vi "Tetra_RxGain.vi"(0 "COMPORT":refnum<visa-resource-name>="COM4", 5 "error in (no error)":errorcluster, 6 "Open Ser(t)":bool, 7 "RXPORT(num)":i32=1 min=1 max=8 step=1, 8 "Close Ser(t)":bool, 9 "GAIN(code)":i32 min=0 max=7 step=1, 11 "REVC(T)":bool=TRUE, 13 "RO(t)":bool) -> (10 "vga(rxport)":string, 12 "gain code(value)":dbl, 14 "comport":refnum<visa-resource-name>="COM4", 16 "Readback (1-4)":i32[](array[numeric]), 19 "error out":errorcluster)   [LabVIEW 2018]
panel:
  out "revcVGA":i32
  out "cmd":string
  out "Success":bool
  out "concatenated string":string
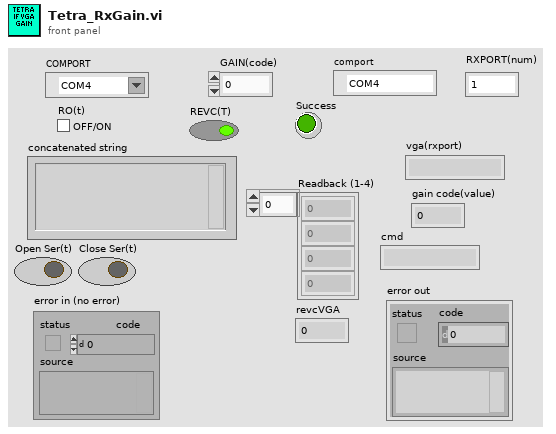
[diagram p1: front panel]
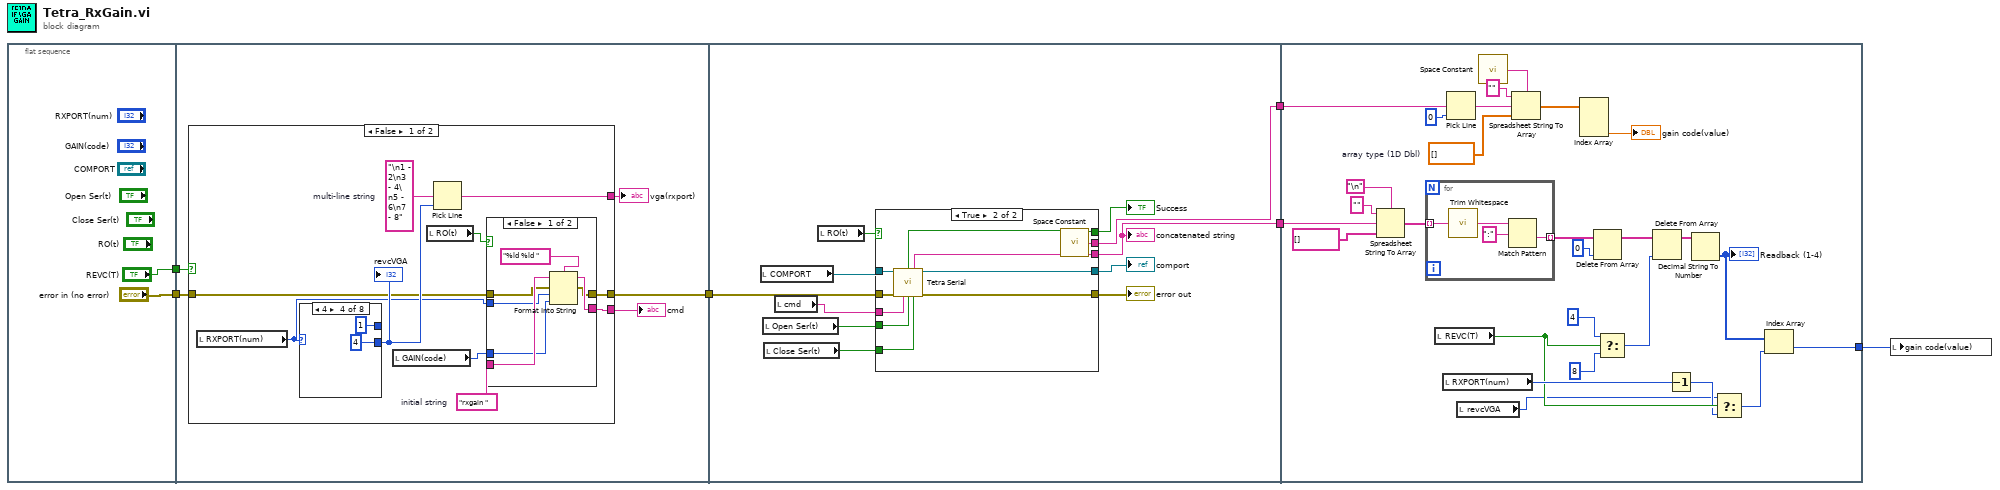
[diagram p0: block diagram]
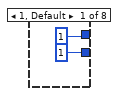
[diagram p3: hidden frame]
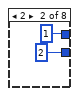
[diagram p4: hidden frame]
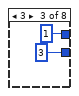
[diagram p5: hidden frame]
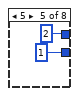
[diagram p6: hidden frame]
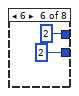
[diagram p7: hidden frame]
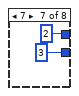
[diagram p8: hidden frame]
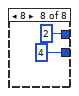
[diagram p9: hidden frame]
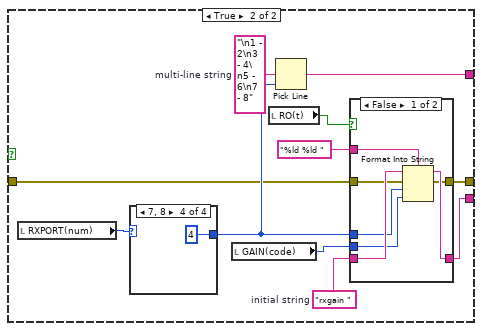
[diagram p10: hidden frame]
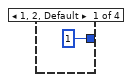
[diagram p12: hidden frame]
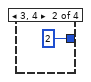
[diagram p13: hidden frame]
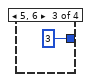
[diagram p14: hidden frame]
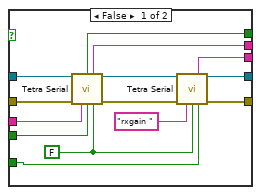
[diagram p15: hidden frame]
diagram:
  n1 = flat-sequence {
    tunnel: ["error in (no error)"] -> w3
    tunnel: ["REVC(T)"] -> w2
    tunnel: [w13] -> w6
    tunnel: w3 -> [w11]
    tunnel: w2 -> [w10]
    tunnel: w6 -> [w79]
    tunnel: [w80] -> w5
    tunnel: [w78] -> w4
    tunnel: w5 -> [w133]
    tunnel: w4 -> [w134]
    tunnel: [w112] -> w1
    frame #0 {
    }
    frame #1 {
      n2 = case shown="False" w10 {
        tunnel: [w23 w59] -> w9
        tunnel: [w22 w58] -> w13
        tunnel: [w19 w54] -> w12
        tunnel: w11 -> [w15 w49]
        frame False {
          w20 = "\n1 - 2\n3 - 4\n5 - 6\n7 - 8"  # multi-line string
          w21 = "rxgain "  # initial string
          n3 = local read "RXPORT(num)"() -> (w14:i32)
          n4 = case shown="4" w14 {
            tunnel: [1 ("RXPORT(num)") 2 ("RXPORT(num)") 3 ("RXPORT(num)") 4 ("RXPORT(num)") 1 ("RXPORT(num)") 2 ("RXPORT(num)") 3 ("RXPORT(num)") 4 ("RXPORT(num)")] -> w18
            tunnel: [1 ("RXPORT(num)") 1 ("RXPORT(num)") 1 ("RXPORT(num)") 1 ("RXPORT(num)") 2 ("RXPORT(num)") 2 ("RXPORT(num)") 2 ("RXPORT(num)") 2 ("RXPORT(num)")] -> _
            frame 1, Default {
            }
            frame 2 {
            }
            frame 3 {
            }
            frame 4 {
            }
            frame 5 {
            }
            frame 6 {
            }
            frame 7 {
            }
            frame 8 {
            }
          }
          "revcVGA" <- w18
          n5 = local read "GAIN(code)"() -> (w16:i32)
          n6 = local read "RO(t)"() -> (w17:bool)
          n7 = Pick Line(multi-line string=w20, line index=w18) -> (output string=w19:string)  [unwired: 1 in]
          n8 = case shown="False" w17 {
            tunnel: [w30 w32] -> w23
            tunnel: w21 -> [w29 w32]
            tunnel: w16 -> [w28 _]
            tunnel: w15 -> [w27 w31]
            tunnel: [w26 w31] -> w22
            tunnel: w14 -> [w24 _]
            frame False {
              n9 = Format Into String(format string="%ld %ld ", initial string=w29, error in=w27, w24, w28) -> (resulting string=w30:string, error out=w26:errorcluster)
            }
            frame True {
            }
          }
        }
        frame True {
          w55 = "\n1 - 2\n3 - 4\n5 - 6\n7 - 8"  # multi-line string
          w56 = "rxgain "  # initial string
          n10 = local read "RXPORT(num)"() -> (w51:i32)
          n11 = case shown="7, 8" w51 {
            tunnel: [1 ("RXPORT(num)") 2 ("RXPORT(num)") 3 ("RXPORT(num)") 4 ("RXPORT(num)")] -> w53
            frame 1, 2, Default {
            }
            frame 3, 4 {
            }
            frame 5, 6 {
            }
            frame 7, 8 {
            }
          }
          n12 = local read "GAIN(code)"() -> (w50:i32)
          n13 = local read "RO(t)"() -> (w52:bool)
          n14 = Pick Line(multi-line string=w55, line index=w53) -> (output string=w54:string)  [unwired: 1 in]
          n15 = case shown="False" w52 {
            tunnel: "%ld %ld " -> [w66 _]
            tunnel: [w65 w68] -> w59
            tunnel: w56 -> [w64 w68]
            tunnel: w50 -> [w63 _]
            tunnel: w53 -> [w62 _]
            tunnel: w49 -> [w61 w67]
            tunnel: [w60 w67] -> w58
            frame False {
              n16 = Format Into String(format string=w66, initial string=w64, error in=w61, w62, w63) -> (resulting string=w65:string, error out=w60:errorcluster)
            }
            frame True {
            }
          }
        }
      }
      "vga(rxport)" <- w12
      "cmd" <- w9
    }
    frame #2 {
      n17 = local read "COMPORT"() -> (w76:refnum<visa-resource-name>)
      n18 = local read "Open Ser(t)"() -> (w75:bool)
      n19 = local read "Close Ser(t)"() -> (w74:bool)
      n20 = local read "cmd"() -> (w73:string)
      n21 = local read "RO(t)"() -> (w77:bool)
      n22 = case shown="True" w77 {
        tunnel: w76 -> [w97 w107]
        tunnel: w73 -> [w96 w106]
        tunnel: [w84 w105] -> w83
        tunnel: [w85 w104] -> w82
        tunnel: [w95 w103] -> w81
        tunnel: w75 -> [w94 w102]
        tunnel: w74 -> [w91 w101]
        tunnel: [w88 w98] -> w80
        tunnel: w79 -> [w93 w100]
        tunnel: [w87 w99] -> w78
        frame False {
          w90 = FALSE ("Close Ser(t)")
          n23 = call "Tetra Serial.vi"("COMPORT"=w97, "error in (no error)"=w93, "Command"=w96, "Open Ser(t)"=w94, "Close Ser(t)"=w90) -> ("Success"=w95:bool, "output"=w88:string, "comport"=w86:refnum<visa-resource-name>, "error out"=w92:errorcluster)  [unwired: 6 in, 1 out]
          n24 = call "Tetra Serial.vi"("COMPORT"=w86, "error in (no error)"=w92, "Command"="rxgain " ("initial string"), "Open Ser(t)"=w90, "Close Ser(t)"=w91) -> ("output"=w87:string, "comport"=w85:refnum<visa-resource-name>, "error out"=w84:errorcluster)  [unwired: 6 in, 2 out]
        }
        frame True {
          n25 = call "Tetra Serial.vi"("COMPORT"=w107, "error in (no error)"=w100, "Command"=w106, "Open Ser(t)"=w102, "Close Ser(t)"=w101) -> ("Success"=w103:bool, "output"=w99:string, "comport"=w104:refnum<visa-resource-name>, "error out"=w105:errorcluster)  [unwired: 6 in, 1 out]
          n26 = call <vilib>:"Space Constant.vi"() -> ("String"=w98:string)
        }
      }
      "comport" <- w82
      "error out" <- w83
      "Success" <- w81
      "concatenated string" <- w78
    }
    frame #3 {
      w130 = dbl[] []  # array type (1D Dbl)
      n27 = Spreadsheet String To Array(delimiter (Tab)="\n", format string="", spreadsheet string=w134, array type (2D Dbl)=string[] []) -> (array=w123:string[])
      n28 = for {
        tunnel: w123 -> [w138] mode=indexing
        tunnel: [w137] -> w122 mode=indexing
        n29 = call <vilib>:"Trim Whitespace.vi"("string"=w138) -> ("trimmed string"=w135:string)  [unwired: 1 in]
        n30 = Match Pattern(string=w135, regular expression=":") -> (after substring=w137:string)  [unwired: 1 in, 3 out]
      }
      n31 = local read "REVC(T)"() -> (w111:bool)
      n32 = local read "RXPORT(num)"() -> (w114:i32)
      n33 = Pick Line(multi-line string=w133, line index=0) -> (output string=w131:string)  [unwired: 1 in]
      n34 = local read "revcVGA"() -> (w108:i32)
      n35 = call <vilib>:"Space Constant.vi"() -> ("String"=w128:string)
      n36 = Spreadsheet String To Array(delimiter (Tab)=w128, format string="", spreadsheet string=w131, array type (2D Dbl)=w130) -> (array=w127:dbl[])
      n37 = Index Array(array=w127) -> (element #3=→"gain code(value)":dbl)  [unwired: 3 in, 2 out]
      n38 = Delete From Array(array=w122, index=0) -> (array with subset deleted=w120:string[])  [unwired: 1 in, 1 out]
      n39 = Select(t=4 ("index"), s=w111, f=8 ("index")) -> (s? t:f=w117:i32)
      n40 = Delete From Array(array=w120, index=w117) -> (array with subset deleted=w119:string[])  [unwired: 1 in, 1 out]
      n41 = Decrement(x=w114) -> (x-1=w110:i32)
      n42 = Decimal String To Number(string=w119) -> (number=w113:i32[])  [unwired: 2 in, 1 out]
      "Readback (1-4)" <- w113
      n43 = Select(t=w108, s=w111, f=w110) -> (s? t:f=w109:i32)
      n44 = Index Array(array=w113, index=w109) -> (element=w112:i32)
    }
  }
  n45 = local write "gain code(value)"(w1) -> ()
